vi "Demo.vi"() -> ()   [LabVIEW 2020, in "Tree Helpers.lvlib" / "LVCLass Tree.lvclass"]
uses:
  LVCLass Tree.lvclass
  File Tree/File Tree.lvclass
  Tag Tree/Tag Tree.lvclass
  LVCLass Tree.lvclass/LVCLass Tree.ctl
panel:
  out "Selected Tags":string[](array[string])
  in  "Tree":string[](tree)
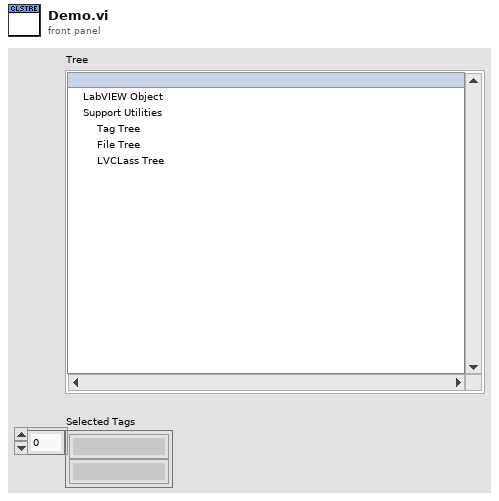
[diagram p1: front panel]
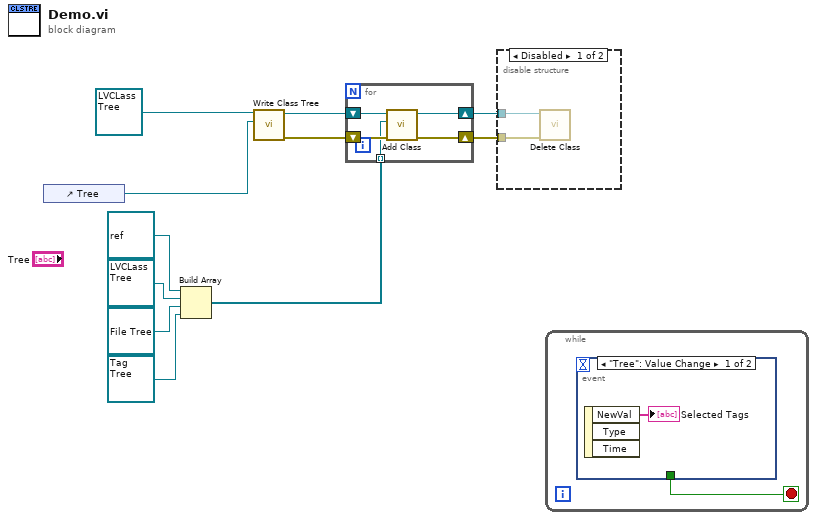
[diagram p0: block diagram]
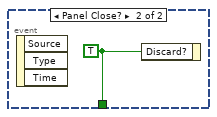
[diagram p3: hidden frame]
diagram:
  n1 = control-ref of="Tree"() -> (w10:refnum<vi>)
  n2 = Build Array(refnum<class> refnum ("LabVIEW Object"), refnum<class "LVCLass Tree.lvclass"> refnum ("Support Utilities.lvlib:Tag Tree.lvclass"), refnum<class "File Tree.lvclass"> refnum ("Support Utilities.lvlib:File Tree.lvclass"), refnum<class "Tag Tree.lvclass"> refnum ("Support Utilities.lvlib:Tag Tree.lvclass")) -> (w5:refnum<class>[])
  n3 = call "Write Class Tree.vi"("Class Tree Reference"=w10, "Tag Tree In"=refnum<class "LVCLass Tree.lvclass"> refnum ("Support Utilities.lvlib:Tag Tree.lvclass")) -> ("error out"=w8:errorcluster, "Tag Tree Out"=w9:refnum<class "LVCLass Tree.lvclass">)  [unwired: 8 in]
  n4 = for {
    tunnel: w5 -> [w12] mode=indexing
    shift-right: [w14] -> w7
    shift-left: w9 -> [w16]
    shift-right: [w13] -> w6
    shift-left: w8 -> [w15]
    n5 = call "Add Class.vi"("error in (no error)"=w15, "Class"=w12, "Tag Tree In"=w16) -> ("error out"=w13:errorcluster, "Tag Tree Out"=w14:refnum<class "LVCLass Tree.lvclass">)  [unwired: 7 in]
  }
  n6 = disable-structure "Diagram Disable Structure" shown="Disabled" {
    disable-tunnel: w7 -> [w18 _]
    disable-tunnel: w6 -> [w17 _]
    frame Disabled {
      n7 = call "Delete Class.vi"("error in (no error)"=w17, "Tag Tree In"=w18) -> ()  [unwired: 8 in, 2 out]
    }
    frame Enabled {
    }
  }
  n8 = while {
    stop <- w19 stop-if-true
    n9 = event shown="[0] \"Tree\": Value Change" {
      selector: _ -> [_ _]
      dyn-events: _ -> [_ _]
      timeout: _ -> [_ _]
      tunnel: [_ w21] -> w19
      event "Tree": Value Change {
        n10 = event-data() -> ("NewVal"=→"Selected Tags":string[])  [unwired: 1 in, 2 out]
      }
      event Panel Close? {
        w21 = TRUE ("Discard?")
        n11 = event-data() -> ()  [unwired: 1 in, 3 out]
        n12 = event-data ("Event Filter Node")("Discard?"=w21) -> ()  [unwired: 1 in, 1 out]
      }
    }
  }
